vi "Create New Worksheet.vi"(8 "error in (no error)":errorcluster, 10 "sheetname":string, 11 "Workbook":refnum<k24>) -> (0 "error out":errorcluster, 3 "worksheet out":refnum<class "worksheet.lvclass">)   [LabVIEW 2017, in "Excel_Specific.lvlib" / "worksheet.lvclass"]
uses:
  worksheet.lvclass
  C:/Users/Neo/Desktop/Dev_Tools_BR/LabVIEW_NPOI/src/lib/NPOI 2.1.1/NPOI.dll
  lib/NPOI 2.1.1/NPOI.dll
  worksheet.lvclass/worksheet.ctl
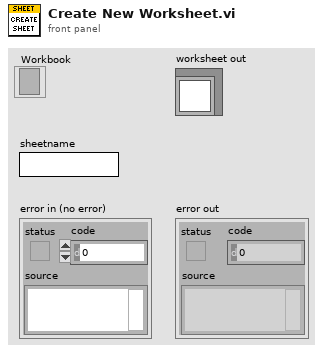
[diagram p1: front panel]
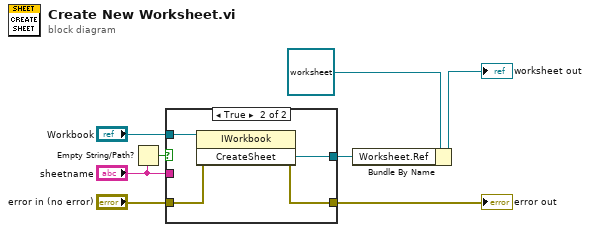
[diagram p0: block diagram]
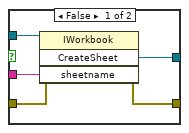
[diagram p2: hidden frame]
diagram:
  n1 = Empty String/Path?(string/path="sheetname") -> (empty?=w3:bool)
  n2 = case shown="True" w3 {
    tunnel: "Workbook" -> [w13 w17]
    tunnel: "sheetname" -> [w12 _]
    tunnel: [w11 w16] -> w1
    tunnel: "error in (no error)" -> [w10 w15]
    tunnel: [w9 w14] -> w7
    frame False {
      n3 = invoke class="IWorkbook" method="CreateSheet"(reference=w13, error in=w10, "sheetname"=w12) -> (error out=w9:errorcluster, "CreateSheet"=w11:refnum<k24>)  [unwired: 1 in, 2 out]
    }
    frame True {
      n4 = invoke class="IWorkbook" method="CreateSheet"(reference=w17, error in=w15) -> (error out=w14:errorcluster, "CreateSheet"=w16:refnum<k24>)  [unwired: 1 in, 1 out]
    }
  }
  "error out" <- w7
  n5 = Bundle By Name(cluster=refnum<class "worksheet.lvclass"> refnum ("worksheet in"), "Worksheet.Ref"=w1) -> (→"worksheet out":refnum<class "worksheet.lvclass">)
